vi "Compile Program.vi"(8 "error in (no error)":errorcluster, 9 "OpenCL Source Code":string, 11 "Device In in":T2) -> (0 "error out":errorcluster, 1 "OpenCL Source Code Out":string, 2 "Program Handle":T1, 3 "Device Out":T2)   [LabVIEW 2012, in "OpenCLV x64.lvlib"]
doc: "Compiles a program that has already been loaded as a string. Only reports that the OpenCL program did or did not compile, not the specific errors."
uses:
  OpenCLV x64.lvlib
  Controls/Device ID.ctl
  Controls/Program Handle.ctl
  Error Checking/Add Error Functional Global.vi
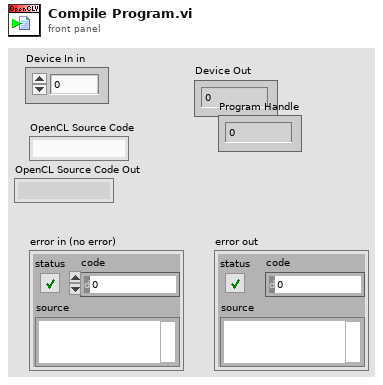
[diagram p1: front panel]
types:
  T1 = typedef "OpenCLV x64.lvlib/Program Handle.ctl" = u64
  T2 = typedef "OpenCLV x64.lvlib/Device ID.ctl" = u64
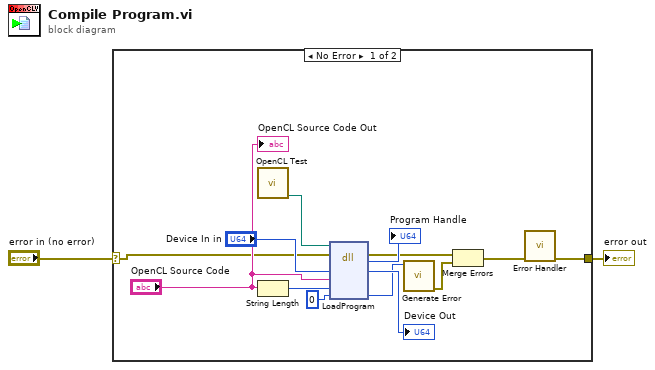
[diagram p0: block diagram]
diagram:
  n1 = case shown="No Error" "error in (no error)" {
    selector: "error in (no error)" -> [w3 w16]
    tunnel: [w7 w16] -> w2
    frame No Error {
      n2 = call "OpenCL Test.vi"() -> ("DLL To Use"=w8:path)  [unwired: 11 in]
      n3 = String Length(string="OpenCL Source Code") -> (length=w15:i32)
      n4 = dll-call lib="C:/Users/bme-amcelroy-la/Desktop/OpenCLV/trunk/OpenCLV_x64_1.0/OpenCLV_x64.dll" fn="LoadProgram"(path in=w8, error in=w3, "Device In"="Device In in", "Program Source"="OpenCL Source Code", "Size of Source"=w15, "Error"=0) -> (error out=w4:errorcluster, "Program Handle"=→"Program Handle":u64, "Device In"=→"Device Out":u64, "Error"=w10:i32)  [unwired: 3 in, 1 out]
      n5 = call "Generate Error.vi"("Error"=w10) -> ("error out"=w6:errorcluster)  [unwired: 10 in]
      n6 = Merge Errors(w4, w6) -> (w5:errorcluster)
      n7 = call-poly "Error Handler.vi"("Error In"=w5) -> ("Error Out"=w7:errorcluster)  [unwired: 10 in]
      "OpenCL Source Code Out" <- "OpenCL Source Code"
    }
    frame Error {
    }
  }
  "error out" <- w2
